vi "Login.vi"(0 "Connection In":refnum<k7>, 1 "error in":errorcluster) -> (2 "Not empty?":bool, 3 "error out":errorcluster, 4 "Connection Out":refnum<k7>, 5 "UserId":string, 6 "Name":string, 7 "Role":string)   [LabVIEW 2022 SP3]
panel:
  out "Password":string
  out "Username":string
  in  "Login":bool
  in  "Cancel":bool
  in  "Cluster":cluster{"Username":string, "Password":string}
  # "Login"
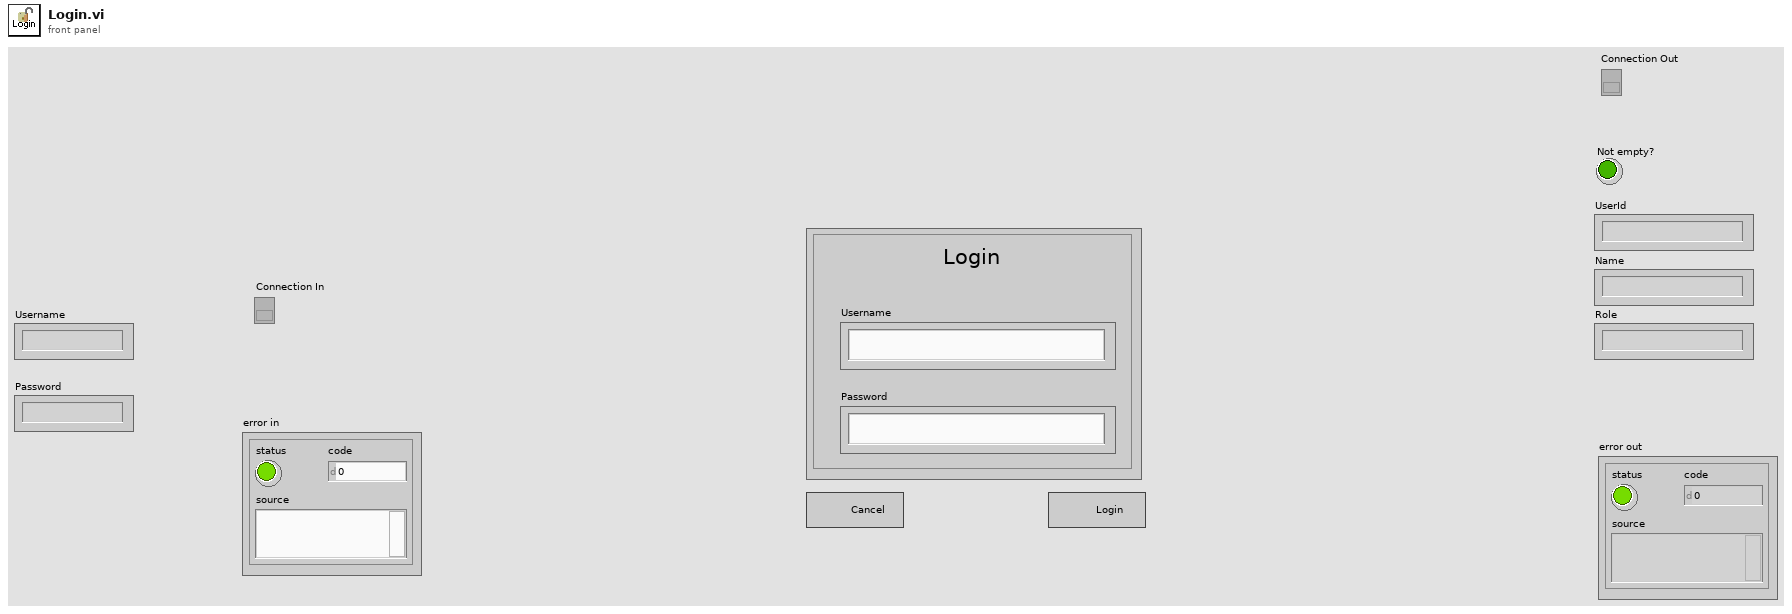
[diagram p1: front panel]
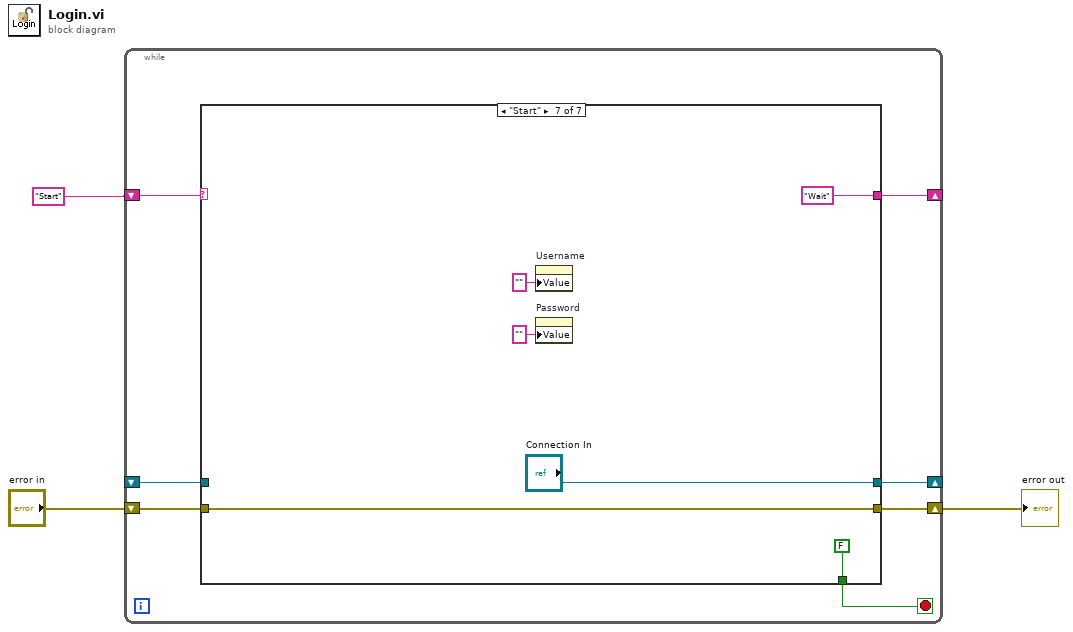
[diagram p0: block diagram]
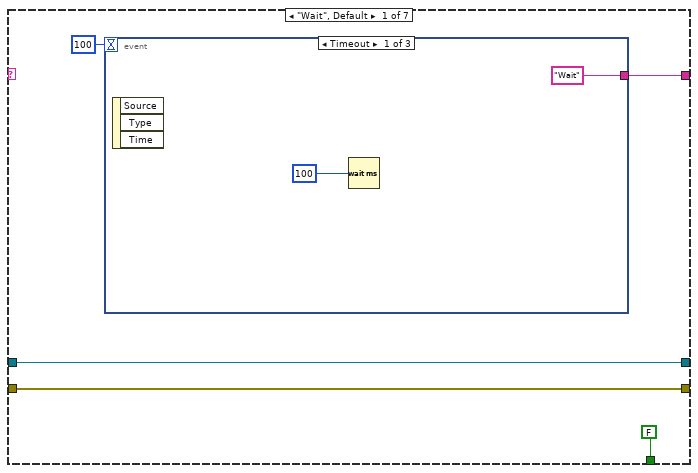
[diagram p2: hidden frame]
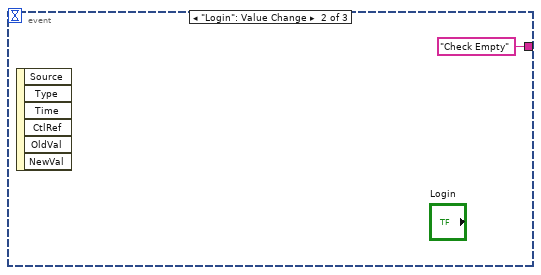
[diagram p3: hidden frame]
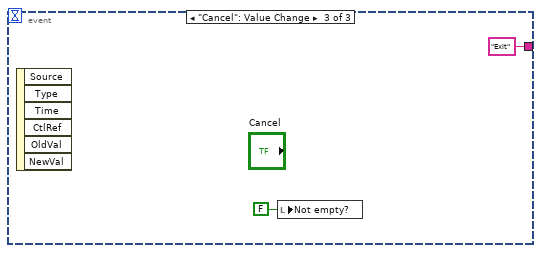
[diagram p4: hidden frame]
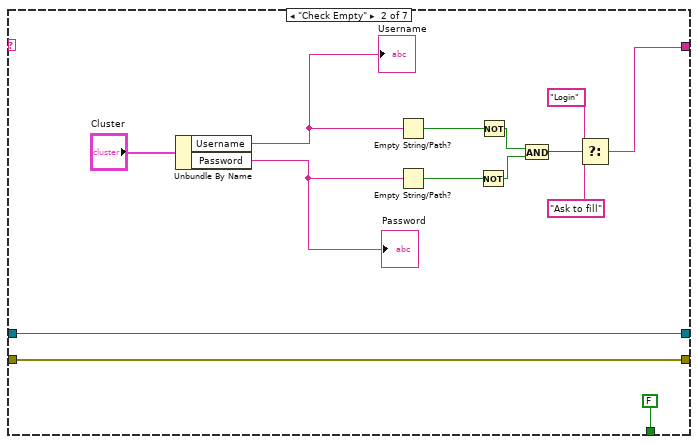
[diagram p5: hidden frame]
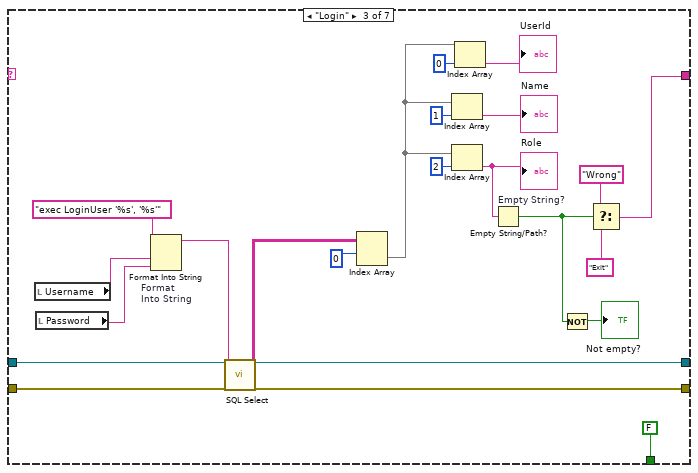
[diagram p6: hidden frame]
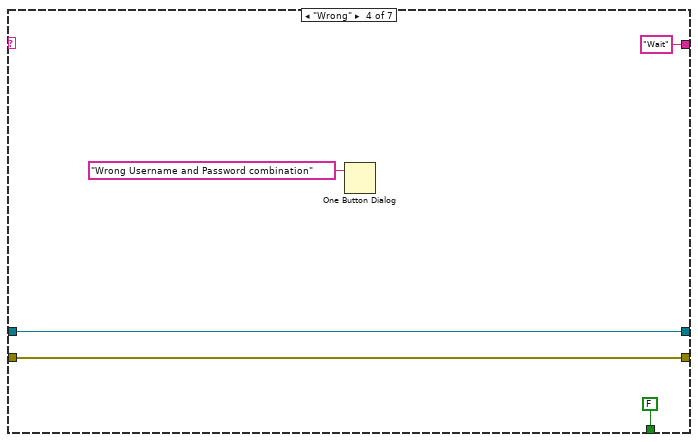
[diagram p7: hidden frame]
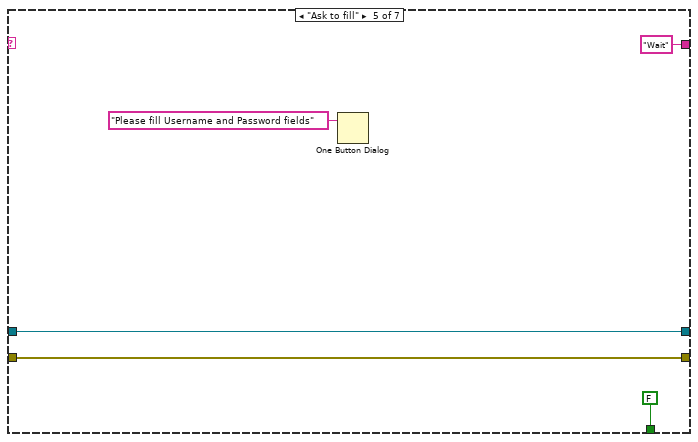
[diagram p8: hidden frame]
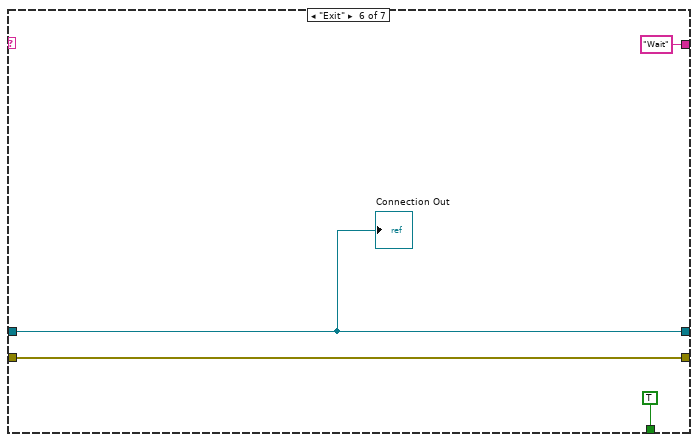
[diagram p9: hidden frame]
diagram:
  n1 = while {
    shift-right: [w9] -> _
    shift-left: "Start" -> [w10]
    shift-right: [w6] -> w1
    shift-left: "error in" -> [w7]
    shift-right: [w5] -> _
    shift-left: _ -> [w4]
    stop <- w8 stop-if-true
    n2 = case shown="\"Start\"" w10 {
      tunnel: [w14 w28 w41 "Wait" ("f") "Wait" ("f") "Wait" "Wait"] -> w9
      tunnel: [FALSE FALSE FALSE FALSE FALSE TRUE FALSE] -> w8
      tunnel: w7 -> [w12 w22 w40 w59 w65 w69 w75]
      tunnel: [w12 w22 w37 w59 w65 w69 w75] -> w6
      tunnel: [w11 w21 w38 w58 w63 w68 "Connection In"] -> w5
      tunnel: w4 -> [w11 w21 w39 w58 w63 w68 _]
      frame "Wait", Default {
        n3 = event shown="[0] Timeout" {
          selector: _ -> [_ _ _]
          dyn-events: _ -> [_ _ _]
          timeout: 100 -> [_ _ _]
          tunnel: ["Wait" "Check Empty" "Exit"] -> w14
          event Timeout {
            n4 = event-data() -> ()  [unwired: 1 in, 3 out]
            n5 = Wait (ms)(milliseconds to wait=u32 100) -> ()  [unwired: 1 out]
          }
          event "Login": Value Change {
            n6 = event-data() -> ()  [unwired: 1 in, 6 out]
          }
          event "Cancel": Value Change {
            n7 = event-data() -> ()  [unwired: 1 in, 6 out]
            n8 = local write "Not empty?"(FALSE ("Not empty?")) -> ()
          }
        }
      }
      frame "Check Empty" {
        n9 = Unbundle By Name("Cluster") -> ("Username"=w33:string, "Password"=w32:string)
        "Username" <- w33
        "Password" <- w32
        n10 = Empty String/Path?(string/path=w33) -> (empty?=w25:bool)
        n11 = Empty String/Path?(string/path=w32) -> (empty?=w24:bool)
        n12 = Not(x=w24) -> (.not. x?=w23:bool)
        n13 = Not(x=w25) -> (.not. x?=w26:bool)
        n14 = And(x=w26, y=w23) -> (x .and. y?=w31:bool)
        n15 = Select(t="Login", s=w31, f="Ask to fill") -> (s? t:f=w28:string)
      }
      frame "Login" {
        n16 = local read "Username"() -> (w55:string)
        n17 = local read "Password"() -> (w54:string)
        n18 = Format Into String "Format \nInto String"(format string="exec LoginUser '%s', '%s'", w55, w54) -> (resulting string=w57:string)  [unwired: 2 in, 1 out]
        n19 = call <vilib>:"SQL Select.vi"("Connection In"=w39, "SQL Query"=w57, "Error in (no error)"=w40) -> ("Connection Out"=w38:refnum<k7>, "Data"=w52:string[][], "Error out"=w37:errorcluster)  [unwired: 14 in]
        n20 = Index Array(array=w52, index (row)=0) -> (element=w45:string[])  [unwired: 1 in]
        n21 = Index Array(array=w45, index=1) -> (element=→"Name":string)
        n22 = Index Array(array=w45, index=2) -> (element=w44:string)
        "Role" <- w44
        n23 = Index Array(array=w45, index=0) -> (element=→"UserId":string)
        n24 = Empty String/Path? "Empty String?"(string/path=w44) -> (empty?=w35:bool)
        n25 = Not(x=w35) -> (.not. x?=→"Not empty?":bool)
        n26 = Select(t="Wrong", s=w35, f="Exit") -> (s? t:f=w41:string)
      }
      frame "Wrong" {
        n27 = One Button Dialog(message="Wrong Username and Password combination") -> ()  [unwired: 1 in, 1 out]
      }
      frame "Ask to fill" {
        n28 = One Button Dialog(message="Please fill Username and Password fields") -> ()  [unwired: 1 in, 1 out]
      }
      frame "Exit" {
        "Connection Out" <- w68
      }
      frame "Start" {
        n29 = property on="Username" class="Str"("Value"="") -> ()  [unwired: 2 in, 2 out]
        n30 = property on="Password" class="Str"("Value"="") -> ()  [unwired: 2 in, 2 out]
      }
    }
  }
  "error out" <- w1
